vi "Output Control.vi"(7 "Communication Address (0)":i16 max=254 format="%x", 8 "error in (no error)":errorcluster, 10 "Enable Output Terminals (F: Off)":bool, 11 "VISA resource name":refnum<visa-resource-name>) -> (0 "error out":errorcluster, 3 "VISA resource name out":refnum<visa-resource-name>)   [LabVIEW 2015, in "BK Precision 178XB Series.lvlib"]
doc: "This VI controls the output terminal of the power supply. If <b>Enable Output Terminals</b> are On, it will enable the output terminals. If Off, it will disable them."
uses:
  BK Precision 178XB Series/BK Precision 178XB Series.lvlib
panel:
  # "(c) 2009 B&K PRECISION CORPORATION.  ALL RIGHTS RESERVED."
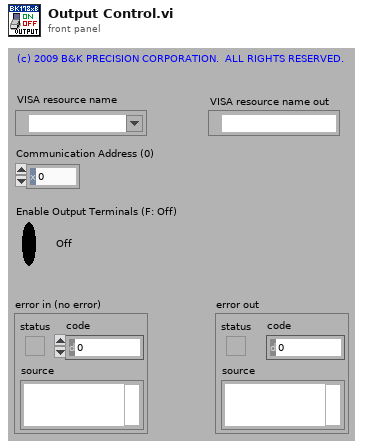
[diagram p1: front panel]
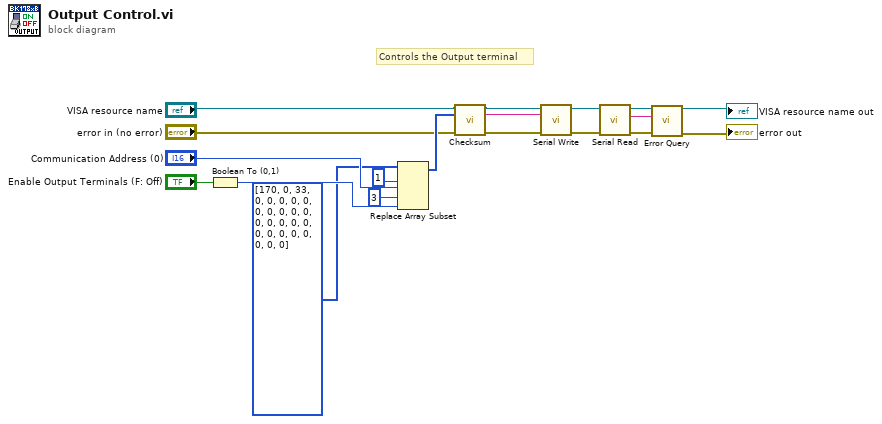
[diagram p0: block diagram]
diagram:
  # "Controls the Output terminal"
  n1 = Boolean To (0,1)(Boolean="Enable Output Terminals (F: Off)") -> (0, 1=w3:i16)
  n2 = Replace Array Subset(array=i16[] [170, 0, 33, 0, 0, 0, 0, 0, 0, 0, 0, 0, 0, 0, 0, 0, 0, 0, 0, 0, 0, 0, 0, 0, 0, 0], new element #1="Communication Address (0)", index #1=1 ("index"), new element #2=w3, index #2=3 ("index")) -> (w11:i16[])
  n3 = call "Checksum.vi"("VISA resource name"="VISA resource name", "Command Frame Array"=w11, "error in (no error)"="error in (no error)") -> ("VISA resource name out"=w8:refnum<visa-resource-name>, "Output String"=w1:string, "error out"=w7:errorcluster)  [unwired: 8 in, 2 out]
  n4 = call "Serial Write.vi"("error in (no error)"=w7, "Input Command Frame"=w1, "VISA resource name"=w8) -> ("error out"=w18:errorcluster, "VISA resource name out"=w17:refnum<visa-resource-name>)  [unwired: 6 in, 1 out]
  n5 = call "Serial Read.vi"("error in (no error)"=w18, "VISA resource name"=w17) -> ("error out"=w14:errorcluster, "Read Buffer"=w15:string, "VISA resource name out"=w16:refnum<visa-resource-name>)  [unwired: 7 in]
  n6 = call "Error Query.vi"("VISA resource name"=w16, "Input Read Buffer 1"=w15, "error in (no error)"=w14) -> ("VISA resource name out"=→"VISA resource name out":refnum<visa-resource-name>, "error out"=→"error out":errorcluster)  [unwired: 7 in, 4 out]
